vi "Query Generator ARB Level Offset.vi"(8 "error in (no error)":errorcluster, 9 "Instance (1)":i32=1, 11 "VISA resource name":refnum<visa-resource-name>) -> (0 "error out":errorcluster, 2 "Level Offset":dbl format="%^.3e", 3 "VISA resource name out":refnum<visa-resource-name>)   [LabVIEW 2020, in "Rohde&Schwarz CMXP GPRF.lvlib"]
doc: "Queries the level offset of the loaded waveform file.\n\nAttribute:\nRSCMXPGPRF_ATTR_ARB_FILE_LEVEL_OFFSET\n\nRemote-control command:\nSOURce:GPRF:GEN<i>:ARB:LOFFset?"
uses:
  <instrlib>/Rohde&Schwarz CMXP GPRF/Rohde&Schwarz CMXP GPRF.lvlib
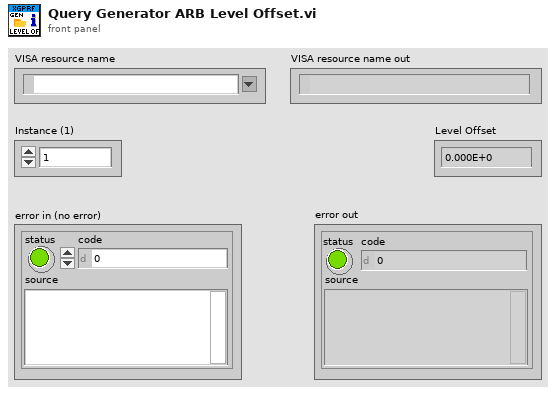
[diagram p1: front panel]
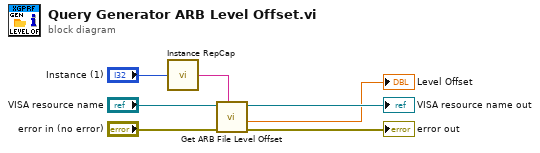
[diagram p0: block diagram]
diagram:
  n1 = call <instrlib>:"Instance RepCap.vi"("Instance in"="Instance (1)") -> ("Instance out"=w7:string)
  n2 = call "Get ARB File Level Offset"("Repeated Capabilities"=w7, "error in (no error)"="error in (no error)", "instrument handle"="VISA resource name") -> ("error out"=→"error out":errorcluster, "ARB File Level Offset"=→"Level Offset":dbl, "instrument handle out"=→"VISA resource name out":refnum<visa-resource-name>)  [unwired: 6 in]
